vi "REST API (GitHub).vi"() -> (0 "error out":errorcluster, 2 "body":string="{\"message\":\"Resource not accessible by personal access token\",\"documentation_url\":\"https://docs.github.com/rest/repos/contents#create-or-update-file-contents\",\"status\":\"403\"}", 3 "headers":string="HTTP/1.1 403 Forbidden\r\nDate: Wed, 09 Apr 2025 08:33:41 GMT\r\nContent-Type: application/json; charset=utf-8\r\nContent-Length: 174\r\nX-GitHub-Media-Type: github.v3; format=json\r\nx-accepted-github-permissions: contents=write; contents=write,workflows=write\r\nx-github-api-version-selected: 2022-11-28\r\nX-RateLimit-Limit: 5000\r\nX-RateLimit-Remaining: 4998\r\nX-RateLimit-Reset: 1744191211\r\nX-RateLimit-Used: 2\r\nX-RateLimit-Resource: core\r\nAccess-Control-Expose-Headers: ETag, Link, Location, Retry-After, X-GitHub-OTP, X-RateLimit-Limit, X-RateLimit-Remaining, X-RateLimit-Used, X-RateLimit-Resource, X-RateLimit-Reset, X-OAuth-Scopes, X-Accepted-OAuth-Scopes, X-Poll-Interval, X-GitHub-Media-Type, X-GitHub-SSO, X-GitHub-Request-Id, Deprecation, Sunset\r\nAccess-Control-Allow-Origin: *\r\nStrict-Transport-Security: max-age=31536000; includeSubdomains; preload\r\nX-Frame-Options: deny\r\nX-Content-Type-Options: nosniff\r\nX-XSS-Protection: 0\r\nReferrer-Policy: origin-when-cross-origin, strict-origin-when-cross-origin\r\nContent-Security-Policy: default-src 'none'\r\nVary: Accept-Encoding, Accept, X-Requested-With\r\nServer: github.com\r\nX-GitHub-Request-Id: F942:2458A5:46A77F:548B41:67F630E5\r\n\r\n")   [LabVIEW 2025]
uses:
  <vilib>/httpClient/PUTBuffer.vi
  <vilib>/httpClient/LabVIEWHTTPClient.lvlib
  <vilib>/JDP Science/JDP Science Common Utilities/Base64/Base64 Support.lvlib
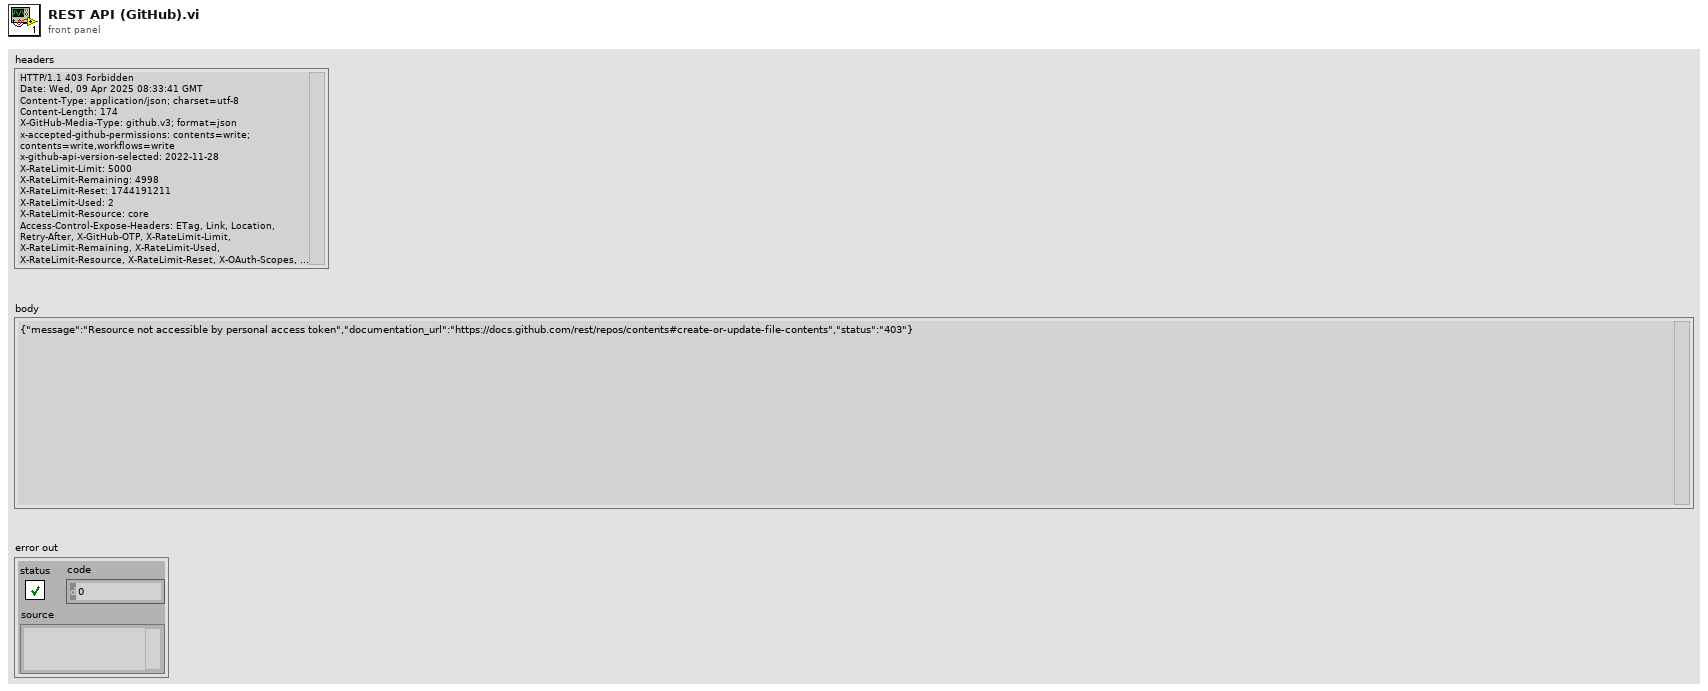
[diagram p1: front panel]
types:
  T1 = typedef "LabVIEWHTTPClient.lvlib/ClientHandle.ctl" = refnum<k1>
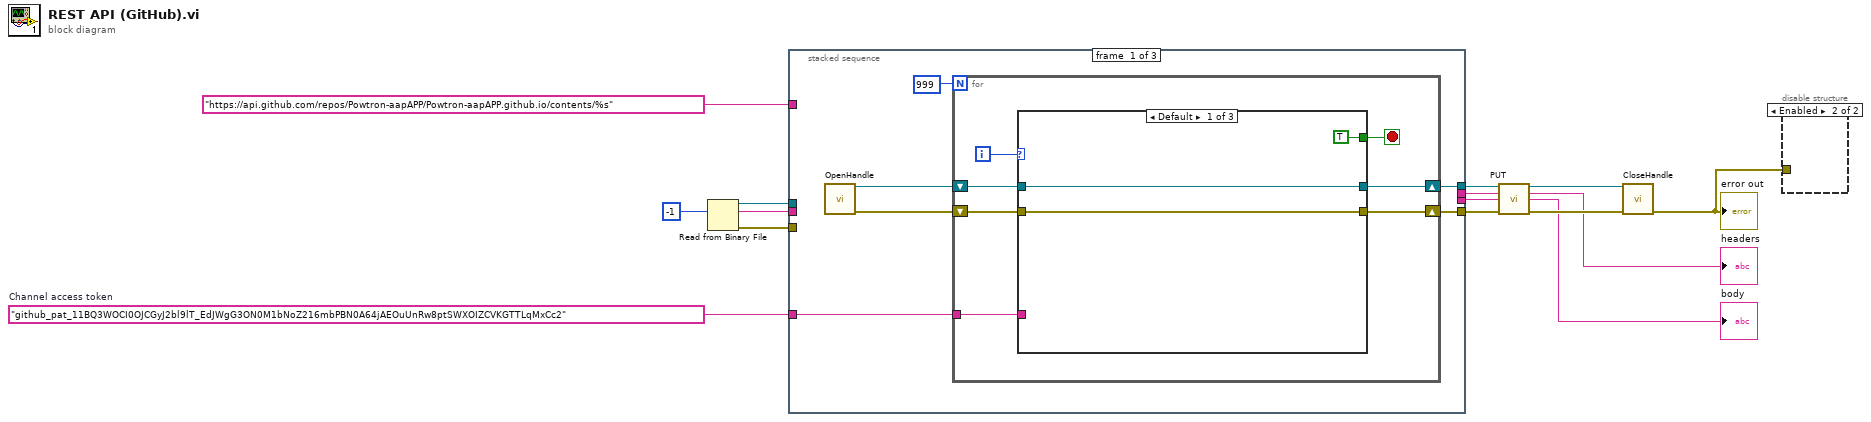
[diagram p0: block diagram]
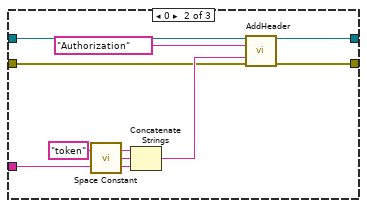
[diagram p2: hidden frame]
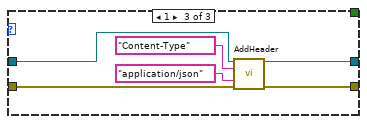
[diagram p3: hidden frame]
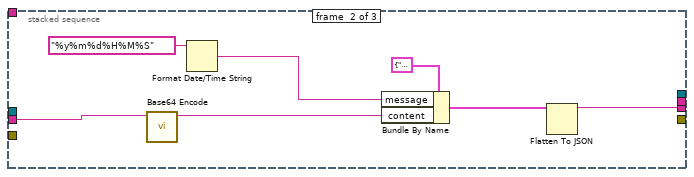
[diagram p4: hidden frame]
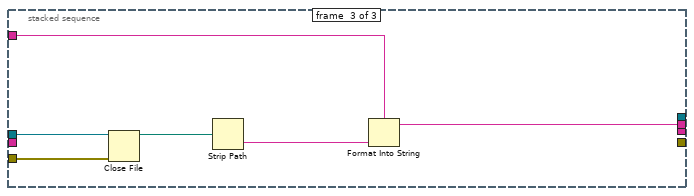
[diagram p5: hidden frame]
diagram:
  w2 = "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"  # Channel access token
  n1 = Read from Binary File(10:-1 ("count (1)")) -> (0:w4:errorcluster, 2:w5:string, 3:w3:refnum<file>)  [unwired: 5 in, 1 out]
  n2 = stacked-sequence {
    tunnel: [w21 _ _] -> w10
    tunnel: [w20 _ _] -> w9
    tunnel: [_ w49 _] -> w7
    tunnel: [_ _ w58] -> w6
    tunnel: w5 -> [_ w48 _]
    tunnel: w4 -> [_ _ w57]
    tunnel: w3 -> [_ _ w56]
    tunnel: w2 -> [w16 _ _]
    tunnel: "https://api.github.com/repos/Powtron-aapAPP/Powtron-aapAPP.github.io/contents/%s" ("url") -> [_ _ w54]
    frame #0 {
      n3 = call <vilib>:"OpenHandle.vi"() -> ("client handle out"=w18:T1, "error out"=w17:errorcluster)  [unwired: 14 in]
      n4 = for {
        N: 999 -> [_]
        shift-right: [w25] -> w21
        shift-left: w18 -> [w27]
        shift-right: [w24] -> w20
        shift-left: w17 -> [w26]
        tunnel: w16 -> [w22]
        i -> [w28]
        stop <- w23 stop-if-true
        n5 = case shown="Default" w28 {
          tunnel: w27 -> [w31 w36 w45]
          tunnel: w26 -> [w30 w34 w43]
          tunnel: [w31 w35 w44] -> w25
          tunnel: [w30 w33 w42] -> w24
          tunnel: [TRUE _ _] -> w23
          tunnel: w22 -> [_ w32 _]
          frame Default {
          }
          frame 0 {
            n6 = call <vilib>:"Space Constant.vi"() -> ("String"=w40:string)
            n7 = Concatenate Strings("token" ("string"), w40, w32) -> (w39:string)
            n8 = call <vilib>:"AddHeader.vi"("client handle"=w36, "header"="Authorization", "value"=w39, "error in (no error)"=w34) -> ("client handle out"=w35:T1, "error out"=w33:errorcluster)  [unwired: 10 in]
          }
          frame 1 {
            n9 = call <vilib>:"AddHeader.vi"("client handle"=w45, "header"="Content-Type", "value"="application/json", "error in (no error)"=w43) -> ("client handle out"=w44:T1, "error out"=w42:errorcluster)  [unwired: 10 in]
          }
        }
      }
    }
    frame #1 {
      n10 = call <vilib>:"Base64 Encode.vi"("String to Encode"=w48) -> ("Base64 Encoded"=w47:string)  [unwired: 10 in]
      n11 = Format Date/Time String(time format string (%c)="%y%m%d%H%M%S") -> (date/time string=w53:string)  [unwired: 2 in]
      n12 = Bundle By Name(cluster=cluster{"message":string, "content":string} {"message"="", "content"=""} ("Cluster"), "message"=w53, "content"=w47) -> (w52:cluster{"message":string, "content":string})
      n13 = Flatten To JSON(anything=w52) -> (JSON string=w49:string)  [unwired: 2 in, 1 out]
    }
    frame #2 {
      n14 = Close File(refnum=w56, error in=w57) -> (path=w55:path)  [unwired: 1 out]
      n15 = Strip Path(path=w55) -> (name=w59:string)  [unwired: 1 out]
      n16 = Format Into String(format string=w54, w59) -> (resulting string=w58:string)  [unwired: 2 in, 1 out]
    }
  }
  n17 = call-poly <vilib>:"PUT.vi"("client handle"=w10, "url"=w6, "buffer"=w7, "error in (no error)"=w9) -> ("client handle out"=w15:T1, "headers"=→"headers":string, "body"=→"body":string, "error out"=w14:errorcluster)  [unwired: 8 in]
  n18 = call <vilib>:"CloseHandle.vi"("client handle"=w15, "error in (no error)"=w14) -> ("error out"=w11:errorcluster)  [unwired: 13 in]
  "error out" <- w11
  n19 = disable-structure shown="Enabled" {
    disable-tunnel: w11 -> [_ _]
    frame Disabled {
    }
    frame Enabled {
    }
  }
